vi "Checksum_compare.vi"(1 "Byte Array":i16[](array[numeric]) format="%.0x") -> (0 "Checksum <>?":bool)   [LabVIEW 2019]
doc: "This vi calculates check sum of received command and compares it with the check sum byte of same received command."
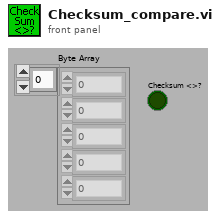
[diagram p1: front panel]
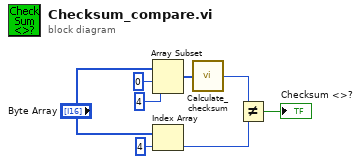
[diagram p0: block diagram]
diagram:
  n1 = Array Subset(array="Byte Array", index=0 ("Array Index"), length=4 ("Array Length")) -> (w5:i16[])
  n2 = Index Array(array="Byte Array", index=4 ("Index")) -> (element=w2:i16)
  n3 = call "Calculate_checksum.vi"("Data"=w5) -> ("Checksum"=w3:i32)
  n4 = Not Equal?(x=w3, y=w2) -> (x != y?=→"Checksum <>?":bool)
